vi "OAT Error Information.vi"(7 "error code":i32) -> (0 "error out":errorcluster)   [LabVIEW 2017]
panel:
  # "Error Information"
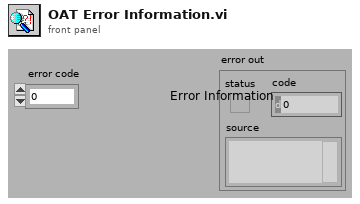
[diagram p1: front panel]
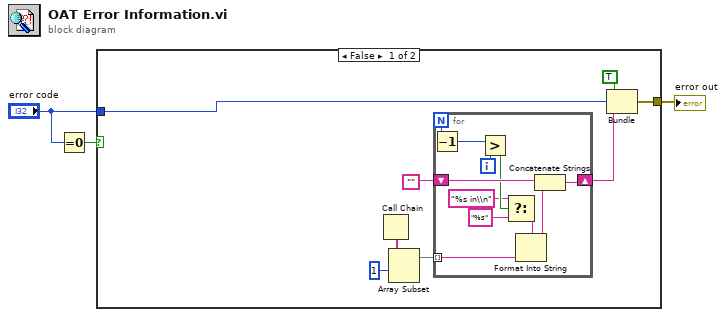
[diagram p0: block diagram]
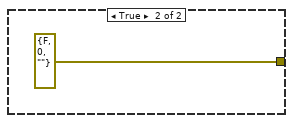
[diagram p2: hidden frame]
diagram:
  n1 = Equal To 0?(x="error code") -> (x = 0?=w3:bool)
  n2 = case shown="False" w3 {
    tunnel: "error code" -> [w4 _]
    tunnel: [w5 errorcluster {"status"=FALSE, "code"=0, "source"=""} ("error out")] -> w1
    frame False {
      n3 = Call Chain() -> (call chain=w8:string[])
      n4 = Array Subset(array=w8, index=1) -> (w9:string[])  [unwired: 1 in]
      n5 = for {
        N -> [w17]
        shift-right: [w21] -> w6
        shift-left: "" -> [w22]
        tunnel: w9 -> [w15] mode=indexing
        i -> [w16]
        n6 = Decrement(x=w17) -> (x-1=w18:i32)
        n7 = Greater?(x=w18, y=w16) -> (0:w19:bool)
        n8 = Select(t="%s in\\n", s=w19, f="%s") -> (s? t:f=w12:string)
        n9 = Format Into String(format string=w12, w15) -> (resulting string=w20:string)  [unwired: 2 in, 1 out]
        n10 = Concatenate Strings(w22, w20) -> (w21:string)
      }
      n11 = Bundle(TRUE, "error code"=w4, w6) -> (w5:cluster{bool, "error code":i32, string})  [unwired: 1 in]
    }
    frame True {
    }
  }
  "error out" <- w1
